vi "Flush Spy Queue.vi"(8 "error in (no error)":errorcluster, 11 "Mock Log Handler in":refnum<class "Mock Log Handler.lvclass">) -> (0 "error out":errorcluster, 2 "remaining elements":T1[](array[typedef]), 3 "Mock Log Handler out":refnum<class "Mock Log Handler.lvclass">)   [LabVIEW 2020, in "Mock Log Handler.lvclass"]
uses:
  Mock Log Handler.lvclass
  Private/Log Entry.ctl
  Mock Log Handler.lvclass/Mock Log Handler.ctl
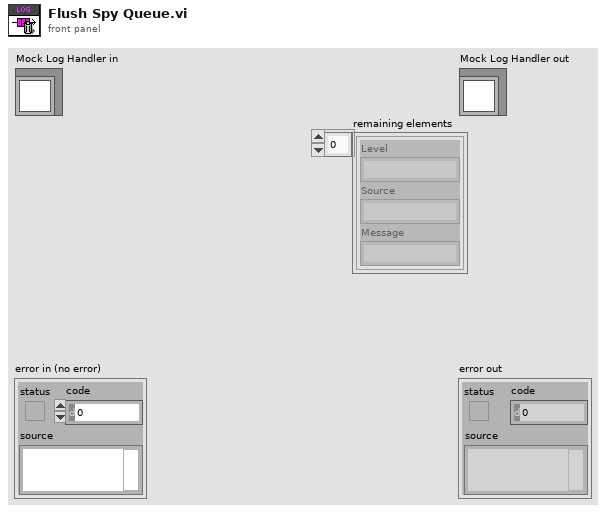
[diagram p1: front panel]
types:
  T1 = typedef "Mock Log Handler.lvclass/Log Entry.ctl" = cluster{"Level":string, "Source":string, "Message":string}
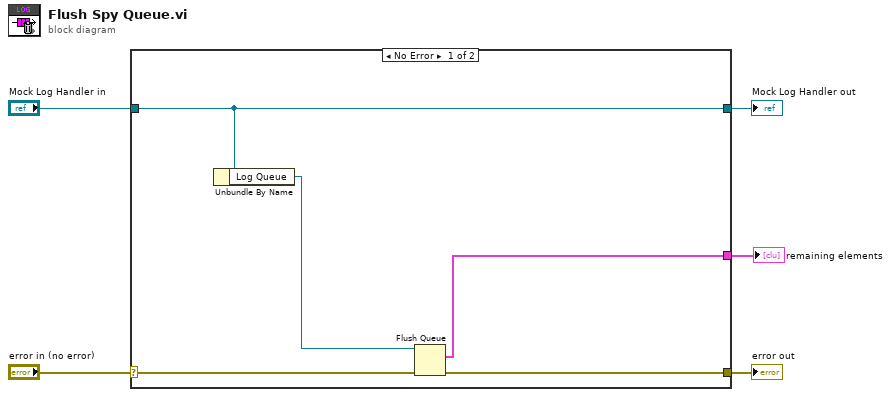
[diagram p0: block diagram]
diagram:
  n1 = case shown="No Error" "error in (no error)" {
    selector: "error in (no error)" -> [w10 w12]
    tunnel: [w8 w12] -> w4
    tunnel: [w9 w11] -> w2
    tunnel: "Mock Log Handler in" -> [w9 w11]
    tunnel: [w6 _] -> w1
    frame No Error {
      n2 = Unbundle By Name(w9) -> ("Log Queue"=w7:refnum<queue>)
      n3 = Flush Queue(queue=w7, error in (no error)=w10) -> (remaining elements=w6:T1[], error out=w8:errorcluster)  [unwired: 1 out]
    }
    frame Error {
    }
  }
  "error out" <- w4
  "Mock Log Handler out" <- w2
  "remaining elements" <- w1
